vi "Diff Configuration.vi"(8 "error in":errorcluster, 10 "configuration new":T4[](array[typedef]), 11 "configuration old":T4[](array[typedef])) -> (0 "error out":errorcluster, 3 "configuration diff":T1[](array[typedef]))   [LabVIEW 2020, in "AIM MIL-STD-1553 System Explorer.lvlib" / "Implementation.lvlib" / "Refresh.lvlib"]
uses:
  Refresh.lvlib
  Change Type.ctl
  Symbols.ctl
  MCL Row.ctl
  Scripting/Constants.vi
  Scripting/AIM MIL-STD-1553 Scripting.lvlib
  Shared/Address.ctl
  Shared/Message Type.ctl
  Shared/Terminal Endpoint.ctl
  Shared/Parameter Definition.ctl
  Shared/Message Definition.ctl
  Shared/1553 Channel.ctl
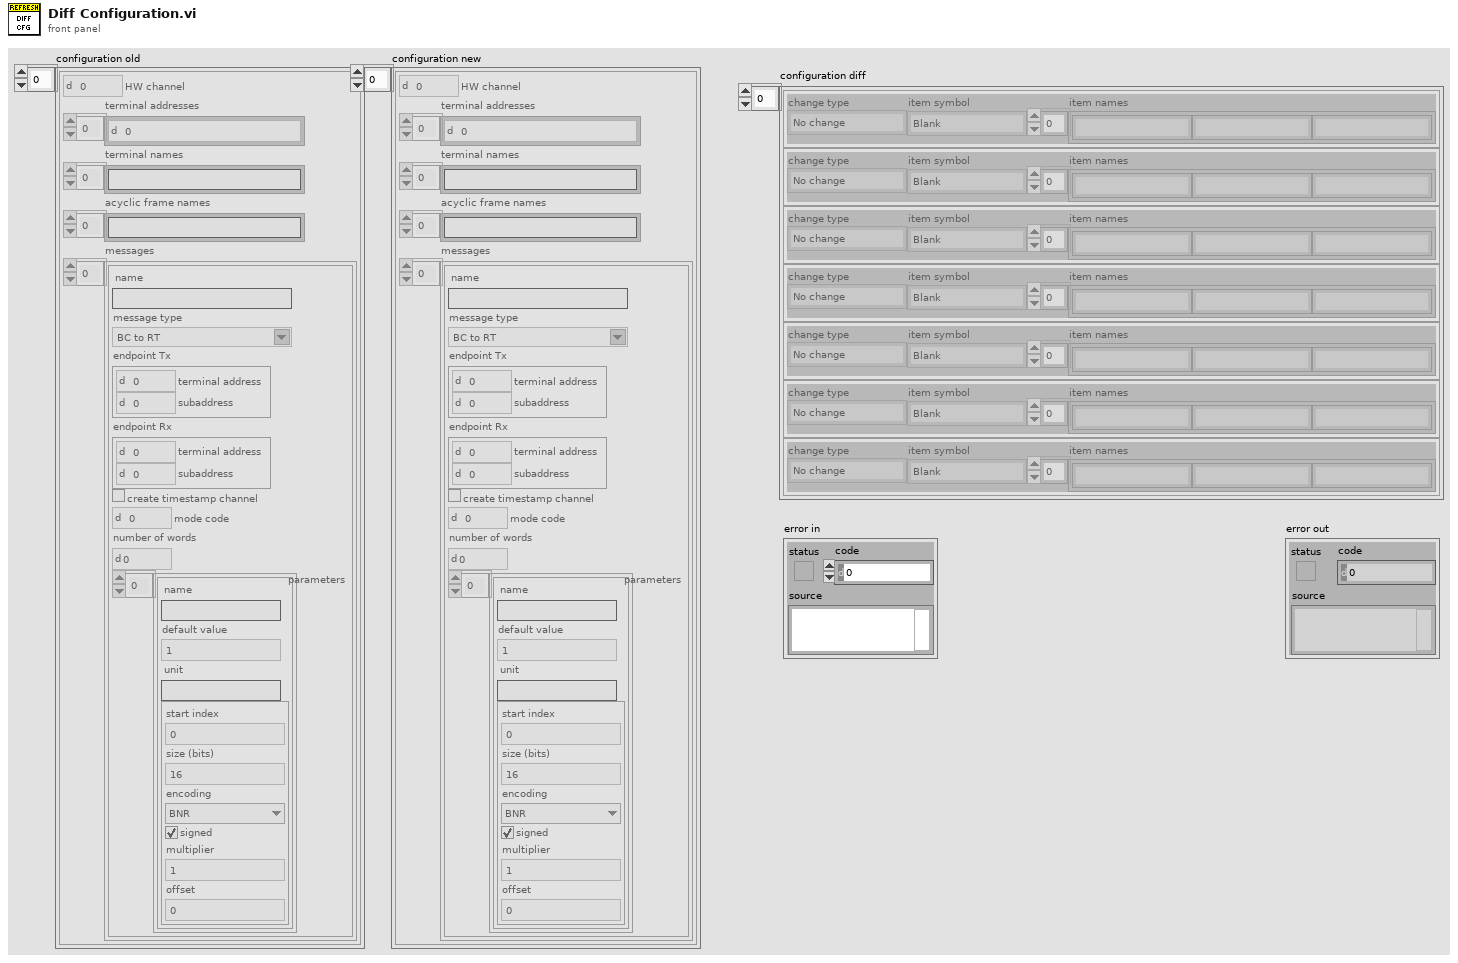
[diagram p1: front panel]
types:
  T1 = typedef "AIM MIL-STD-1553 System Explorer.lvlib/Implementation.lvlib/Refresh.lvlib/MCL Row.ctl" = cluster{"change type":T2, "item symbol":T3, "item names":string[]}
  T2 = typedef "AIM MIL-STD-1553 System Explorer.lvlib/Implementation.lvlib/Refresh.lvlib/Change Type.ctl" = enum16{"No change", "Modify", "Add", "Remove"}
  T3 = typedef "AIM MIL-STD-1553 System Explorer.lvlib/Implementation.lvlib/Refresh.lvlib/Symbols.ctl" = enum16{"Blank", "MIL-STD-1553", "Port", "Remote Terminal", "Subaddress", "Bus Controller", "Acyclic Frame", "Mode Code", "Message", "Parameter", "Item"}
  T4 = typedef "1553 Channel.ctl" = cluster{"HW channel":u16, "terminal addresses":T5[], "terminal names":string[], "acyclic frame names":string[], "messages":T6[]}
  T5 = typedef "Address.ctl" = u16
  T6 = typedef "Message Definition.ctl" = cluster{"name":string, "message type":T7, "endpoint Tx":T8, "endpoint Rx":T8, "create timestamp channel":bool, "mode code":u16, "number of words":u16, "parameters":cluster{"name":string, "default value":dbl, "unit":string, "parameter definition":T9}[]}
  T7 = typedef "Message Type.ctl" = string
  T8 = typedef "Terminal Endpoint.ctl" = cluster{"terminal address":T5, "subaddress":T5}
  T9 = typedef "Parameter Definition.ctl" = cluster{"start index":i32, "size (bits)":i32, "encoding":enum16{"BNR", "BCD", "Discrete"}, "signed":bool, "multiplier":dbl, "offset":dbl}
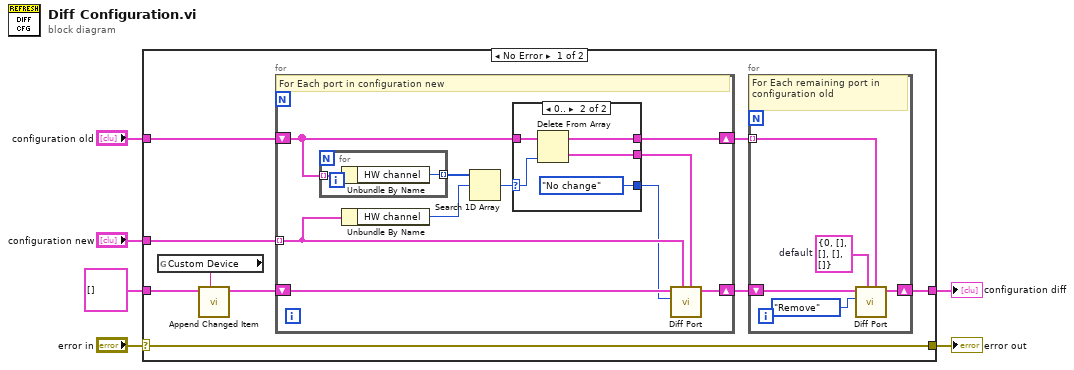
[diagram p0: block diagram]
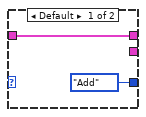
[diagram p2: hidden frame]
diagram:
  n1 = case shown="No Error" "error in" {
    selector: "error in" -> [w14 w40]
    tunnel: T1[] [] -> [w15 w41]
    tunnel: [w8 w41] -> w5
    tunnel: [w14 w40] -> w3
    tunnel: "configuration old" -> [w13 _]
    tunnel: "configuration new" -> [w12 _]
    frame No Error {
      n2 = global read "Constants.vi" "Custom Device"() -> (w7:string)
      n3 = call "Append Changed Item.vi"("item name"=w7, "refresh items in"=w15) -> ("refresh items out"=w11:T1[])  [unwired: 8 in, 1 out]
      n4 = for {
        tunnel: w12 -> [w23] mode=indexing
        shift-right: [w27] -> w9
        shift-left: w13 -> [w28]
        shift-right: [w25] -> w10
        shift-left: w11 -> [w22]
        # "For Each port in configuration new"
        n5 = for {
          tunnel: w28 -> [w39] mode=indexing
          tunnel: [w38] -> w30 mode=indexing
          n6 = Unbundle By Name(w39) -> ("HW channel"=w38:u16)
        }
        n7 = Unbundle By Name(w23) -> ("HW channel"=w29:u16)
        n8 = Search 1D Array(1D array=w30, element=w29) -> (index of element=w26:i32)  [unwired: 1 in]
        n9 = case shown="0.." w26 {
          selector: w26 -> [_ w35]
          tunnel: w28 -> [w32 w37]
          tunnel: [w32 w36] -> w27
          tunnel: [_ w34] -> w24
          tunnel: [Change_Type."Add" ("change type") Change_Type."No change" ("change type")] -> w21
          frame Default {
          }
          frame 0.. {
            n10 = Delete From Array(array=w37, index=w35) -> (deleted portion=w34:T4, array with subset deleted=w36:T4[])  [unwired: 1 in]
          }
        }
        n11 = call "Diff Port.vi"("port old"=w24, "port new"=w23, "change type"=w21, "refresh items in"=w22) -> ("refresh items out"=w25:T1[])  [unwired: 7 in]
      }
      n12 = for {
        shift-right: [w18] -> w8
        shift-left: w10 -> [w20]
        tunnel: w9 -> [w17] mode=indexing
        w16 = T4 {"HW channel"=0, "terminal addresses"=[], "terminal names"=[], "acyclic frame names"=[], "messages"=[]}  # default
        # "For Each remaining port in configuration old"
        n13 = call "Diff Port.vi"("port old"=w17, "port new"=w16, "change type"=Change_Type."Remove", "refresh items in"=w20) -> ("refresh items out"=w18:T1[])  [unwired: 7 in]
      }
    }
    frame Error {
    }
  }
  "configuration diff" <- w5
  "error out" <- w3
